vi "Close MeasurementLink Session.vi"(8 "error in":errorcluster, 9 "initialize and close session behavior":T1, 10 "session in":variant, 11 "session factory in":refnum<class "Session Factory.lvclass">) -> (0 "error out":errorcluster)   [LabVIEW 2021, in "NI Session Management niDCPower.lvlib" / "Session Factory.lvclass"]
uses:
  Session Factory.lvclass
  Instrument/ISession Factory/Initialize and Close Session Behavior.ctl
  Instrument/ISession Factory/ISession Factory.lvclass
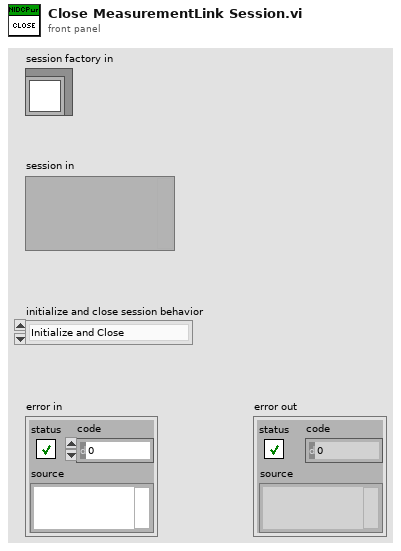
[diagram p1: front panel]
types:
  T1 = typedef "NI Session Management Instrument.lvlib/ISession Factory.lvclass/Initialize and Close Session Behavior.ctl" = enum16{"Initialize and Close", "Attach and Detach", "Initialize and Detach", "Attach and Close"}
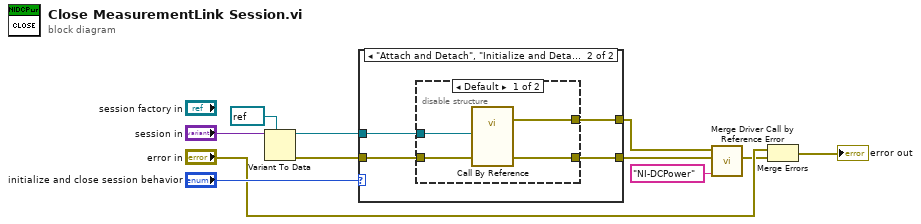
[diagram p0: block diagram]
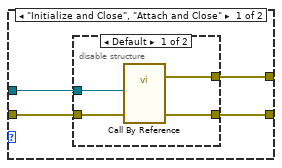
[diagram p2: hidden frame]
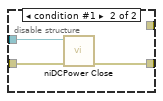
[diagram p3: hidden frame]
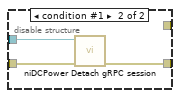
[diagram p4: hidden frame]
diagram:
  n1 = Variant To Data(type=refnum<k15> refnum ("instrument handle"), Variant="session in") -> (data=w7:refnum<k15>, error out=w8:errorcluster)  [unwired: 1 in]
  n2 = case shown="\"Attach and Detach\", \"Initialize and Detach\"" "initialize and close session behavior" {
    tunnel: w8 -> [w15 w26]
    tunnel: w7 -> [w14 w25]
    tunnel: [w13 w24] -> w2
    tunnel: [w12 w23] -> w3
    frame "Initialize and Close", "Attach and Close" {
      n3 = disable-structure shown="Default" {
        disable-tunnel: w15 -> [w19 w22]
        disable-tunnel: w14 -> [w18 w20]
        disable-tunnel: [w17 w21] -> w13
        disable-tunnel: [w16 _] -> w12
        frame condition #0 (active) {
          n4 = call-by-ref "?"("error in (no error)"=w19, "instrument handle"=w18) -> (error out=w16:errorcluster, 0:"error out"=w17:errorcluster)  [unwired: 11 in, 1 out]
        }
        frame condition #1 {
          n5 = call <instrlib>:"niDCPower Close.vi"("error in (no error)"=w22, "instrument handle"=w20) -> ("error out"=w21:errorcluster)  [unwired: 9 in]
        }
      }
    }
    frame "Attach and Detach", "Initialize and Detach" {
      n6 = disable-structure shown="Default" {
        disable-tunnel: w26 -> [w30 w33]
        disable-tunnel: w25 -> [w29 w31]
        disable-tunnel: [w28 w32] -> w24
        disable-tunnel: [w27 _] -> w23
        frame condition #0 (active) {
          n7 = call-by-ref "?"("error in (no error)"=w30, "instrument handle"=w29) -> (error out=w27:errorcluster, 0:"error out"=w28:errorcluster)  [unwired: 11 in, 1 out]
        }
        frame condition #1 {
          n8 = call <instrlib>:"niDCPower Detach gRPC session.vi"("error in (no error)"=w33, "instrument handle"=w31) -> ("error out"=w32:errorcluster)  [unwired: 9 in]
        }
      }
    }
  }
  n9 = call "Merge Driver Call by Reference Error.vi"("driver name"="NI-DCPower", "called vi error"=w2, "call by ref error"=w3) -> ("error out"=w1:errorcluster)  [unwired: 8 in]
  n10 = Merge Errors("error in", w1) -> (→"error out":errorcluster)
